vi "uPolicy_hasPrefix_Set.vi"(8 "error in (no error)":errorcluster, 10 "prefix":string, 11 "hasPrefix in":refnum<class "hasPrefix.lvclass">) -> (0 "error out":errorcluster, 3 "hasPrefix out":refnum<class "hasPrefix.lvclass">)   [LabVIEW 2021, in "uFramework_pack_uPolicy.lvlib" / "hasPrefix.lvclass"]
doc: "Set the prefix of topics to which this policy subscribes."
uses:
  hasPrefix.lvclass
  hasPrefix.lvclass/hasPrefix.ctl
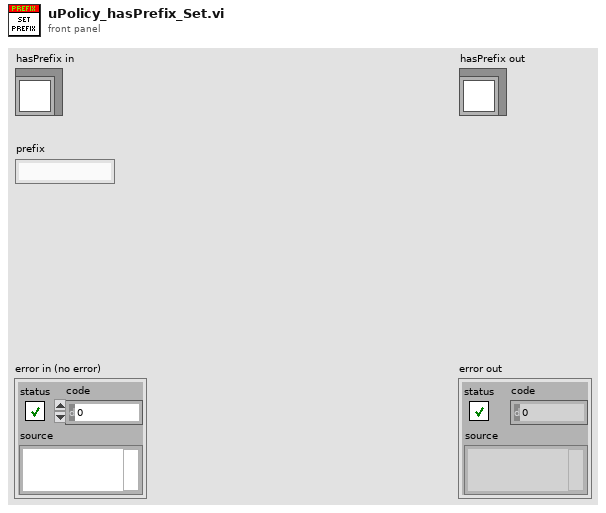
[diagram p1: front panel]
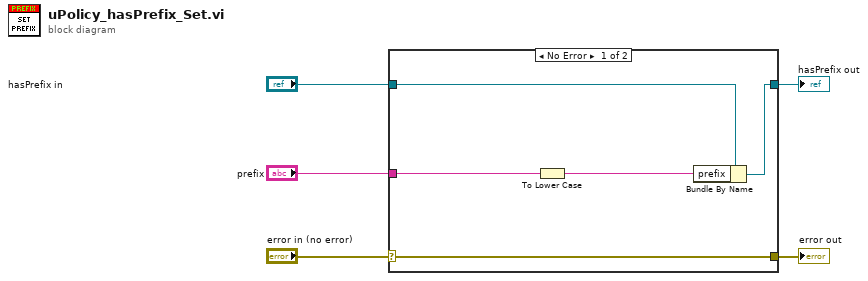
[diagram p0: block diagram]
diagram:
  n1 = case shown="No Error" "error in (no error)" {
    selector: "error in (no error)" -> [w10 w11]
    tunnel: [w10 w11] -> w4
    tunnel: [w8 w12] -> w2
    tunnel: "hasPrefix in" -> [w9 w12]
    tunnel: "prefix" -> [w7 _]
    frame No Error {
      n2 = To Lower Case(string=w7) -> (all lower case string=w6:string)
      n3 = Bundle By Name(cluster=w9, "prefix"=w6) -> (w8:refnum<class "hasPrefix.lvclass">)
    }
    frame Error {
    }
  }
  "error out" <- w4
  "hasPrefix out" <- w2
